vi "RTD_load_preset.vi"(8 "error in":errorcluster, 11 "file path":path) -> (0 "error out":errorcluster, 1 "failed":bool, 2 "successfull":bool, 3 "preset":T1 {"tref" format="%.3f"; "Rref [Ohm]" format="%.3f"; "RTD poly" format="%_6e"})   [LabVIEW 2020]
uses:
  RTD_preset.ctl
  <vilib>/Utility/file.llb/Read From Spreadsheet File (string).vi
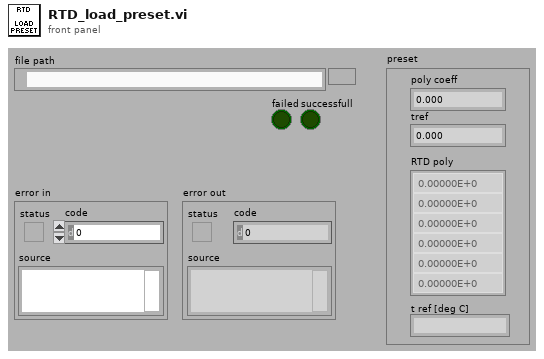
[diagram p1: front panel]
types:
  T1 = typedef "RTD_preset.ctl" = cluster{"Rref [Ohm]":dbl, "tref":dbl, "RTD poly":dbl[], "name":string}
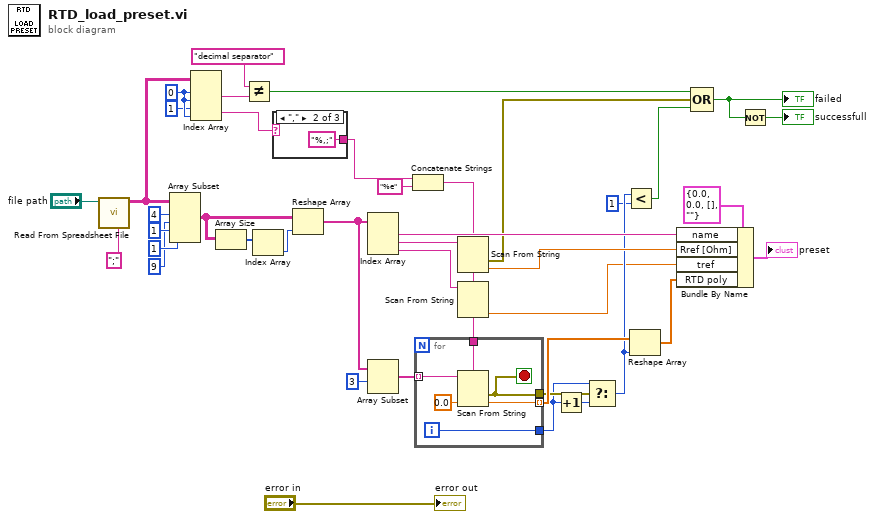
[diagram p0: block diagram]
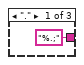
[diagram p2: hidden frame]
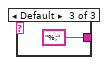
[diagram p3: hidden frame]
diagram:
  w37 = 0 ("index (row)")
  n1 = call-poly <vilib>:"Read From Spreadsheet File.vi"("delimiter (\\t)"=";" ("delimiter (\\t)"), "file path (dialog if empty)"="file path") -> ("all rows"=w28:string[][])  [unwired: 5 in, 4 out]
  n2 = Array Subset(array=w28, index (row)=4 ("index"), length (row)=9 ("length"), index (col)=1 ("index"), length (col)=1 ("length")) -> (w31:string[][])
  n3 = Index Array(array=w28, index (row) #1=w37, index (col) #1=w37, index (row) #2=1 ("disabled index (row)"), index (col) #2=w37) -> (element #1=w39:string, element #2=w35:string)
  n4 = Array Size(array=w31) -> (size(s)=w30:i32[])
  n5 = Not Equal?(x="decimal separator", y=w39) -> (x != y?=w21:bool)
  n6 = Index Array(array=w30) -> (element=w29:i32)  [unwired: 1 in]
  n7 = case shown="\",\"" w35 {
    tunnel: ["%.;" "%,;" "%;"] -> w23
    frame "." {
    }
    frame "," {
    }
    frame Default {
    }
  }
  n8 = Reshape Array(w31, w29) -> (w18:string[])
  n9 = Index Array(array=w18) -> (element #1=w25:string, element #2=w24:string, element #3=w3:string)  [unwired: 3 in]
  n10 = Array Subset(array=w18, index=3) -> (w16:string[])  [unwired: 1 in]
  n11 = Concatenate Strings(w23, "%e" ("string")) -> (w4:string)
  n12 = for {
    tunnel: w16 -> [w49] mode=indexing
    tunnel: w4 -> [w50]
    tunnel: [w48] -> w15 mode=indexing
    tunnel: [w46] -> w12
    tunnel: [w45] -> w14
    i -> [w46]
    stop <- w45 stop-if-true
    n13 = Scan From String(format string=w50, input string=w49, default 1=0.0 ("default value 1")) -> (error out=w45:errorcluster, output 1=w48:dbl)  [unwired: 2 in, 2 out]
  }
  n14 = Scan From String(format string=w4, input string=w24) -> (error out=w20:errorcluster, output 1=w19:dbl)  [unwired: 3 in, 2 out]
  n15 = Scan From String(format string=w4, input string=w3) -> (output 1=w1:dbl)  [unwired: 3 in, 3 out]
  n16 = Increment(x=w12) -> (x+1=w13:i32)
  n17 = Select(t=w12, s=w14, f=w13) -> (s? t:f=w10:i32)
  n18 = Less?(x=w10, y=1) -> (x < y?=w8:bool)
  n19 = Reshape Array(w15, w10) -> (w2:dbl[])
  n20 = Bundle By Name(cluster=T1 {"Rref [Ohm]"=0.0, "tref"=0.0, "RTD poly"=[], "name"=""} ("preset"), "name"=w25, "Rref [Ohm]"=w19, "tref"=w1, "RTD poly"=w2) -> (→"preset":T1)
  n21 = Compound Arithmetic op=OR(w21, w20, w8) -> (w6:bool)
  "failed" <- w6
  n22 = Not(x=w6) -> (.not. x?=→"successfull":bool)
  "error out" <- "error in"
